vi "S2C_FORNAX_Proc_UpdateFornaxGlobal.vi"(8 "Error In":errorcluster, 9 "Values":string[](array[string]), 10 "Keys":string[](array[string]), 11 "Section":string) -> (0 "Error Out":errorcluster)   [LabVIEW 2015]
doc: "Loads the Fornax Command file values into their respective globals."
uses:
  S2C_FORNAX_Proc_Globals.vi
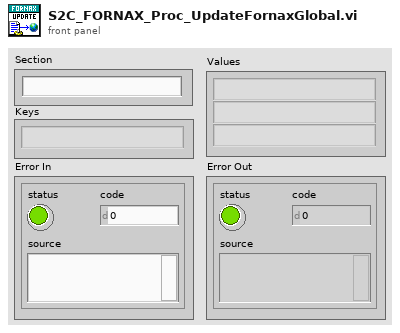
[diagram p1: front panel]
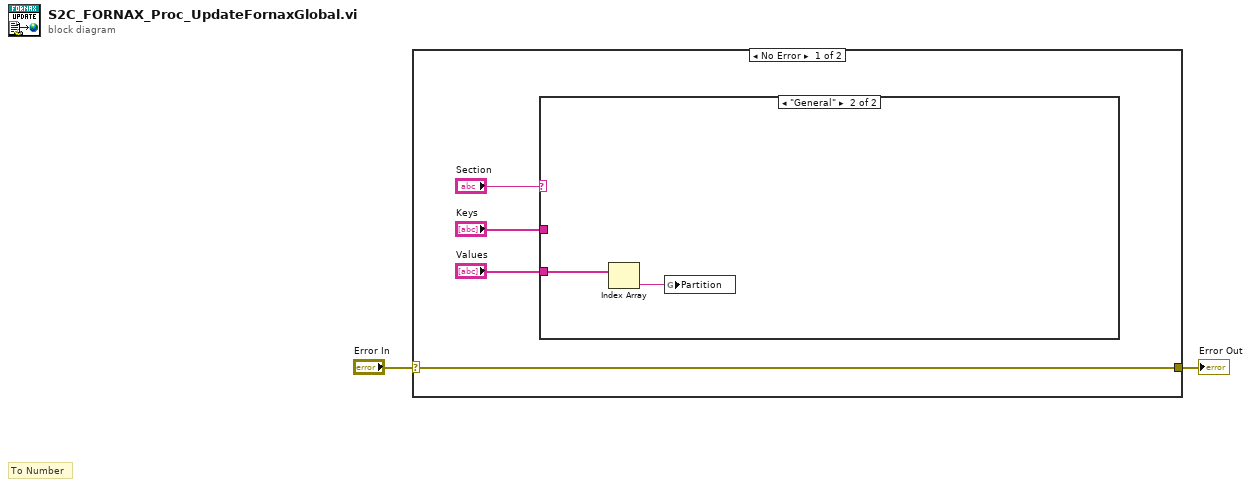
[diagram p0: block diagram]
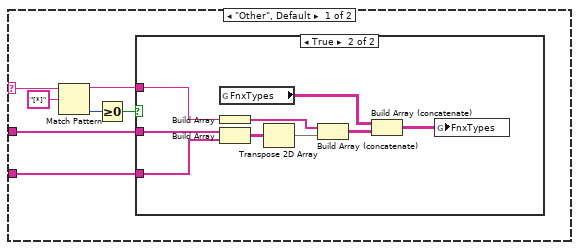
[diagram p2: hidden frame]
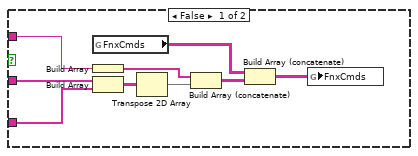
[diagram p3: hidden frame]
diagram:
  # "To Number"
  n1 = case shown="No Error" "Error In" {
    selector: "Error In" -> [w4 w34]
    tunnel: [w4 w34] -> w1
    frame No Error {
      n2 = case shown="\"General\"" "Section" {
        selector: "Section" -> [w7 _]
        tunnel: "Keys" -> [w13 _]
        tunnel: "Values" -> [w12 w33]
        frame "Other", Default {
          n3 = Match Pattern(string=w7, regular expression="[*]") -> (before substring=w10:string, offset past match=w8:i32)  [unwired: 1 in, 2 out]
          n4 = Greater Or Equal To 0?(x=w8) -> (x >= 0?=w9:bool)
          n5 = case shown="True" w9 {
            tunnel: w13 -> [w18 w27]
            tunnel: w12 -> [w17 w26]
            tunnel: w10 -> [w16 w25]
            frame False {
              n6 = global read "S2C_FORNAX_Proc_Globals.vi" "FnxCmds"() -> (w15:string[][][])
              n7 = Build Array(w16) -> (w20:string[])
              n8 = Build Array(w18, w17) -> (w22:string[][])
              n9 = Transpose 2D Array(2D array=w22) -> (transposed array=w21:string[][])
              n10 = Build Array (concatenate)(w20, w21) -> (w19:string[][])
              n11 = Build Array (concatenate)(w15, w19) -> (w14:string[][][])
              n12 = global write "S2C_FORNAX_Proc_Globals.vi" "FnxCmds"(w14) -> ()
            }
            frame True {
              n13 = global read "S2C_FORNAX_Proc_Globals.vi" "FnxTypes"() -> (w24:string[][][])
              n14 = Build Array(w25) -> (w29:string[])
              n15 = Build Array(w27, w26) -> (w31:string[][])
              n16 = Transpose 2D Array(2D array=w31) -> (transposed array=w30:string[][])
              n17 = Build Array (concatenate)(w29, w30) -> (w28:string[][])
              n18 = Build Array (concatenate)(w24, w28) -> (w23:string[][][])
              n19 = global write "S2C_FORNAX_Proc_Globals.vi" "FnxTypes"(w23) -> ()
            }
          }
        }
        frame "General" {
          n20 = Index Array(array=w33) -> (element=w32:string)  [unwired: 1 in]
          n21 = global write "S2C_FORNAX_Proc_Globals.vi" "Partition"(w32) -> ()
        }
      }
    }
    frame Error {
    }
  }
  "Error Out" <- w1
